vi "Phase control (SubVI).vi"() -> ()   [LabVIEW 2018]
uses:
  <vilib>/measure/mamon.llb/Waveform Peak Detection for 1 Chan.vi
  <vilib>/measure/NI_MAPro.lvlib
panel:
  in  "step search":i32=2 caption="Шаг поиска минимума"
  out "pos_xy":cluster{"pos_x":dbl, "pos_y":dbl} caption="Позиция 2D, мм"
  in  "check":bool
  in  "s_search":bool
  in  "n_search":bool
  in  "start_p_s":bool
  in  "start_p_ns":bool
  out "s_done":bool
  out "n_done":bool
  out "n_sel_pos":dbl
  out "s_sel_pos":dbl
  out "n_arr":dbl[](array[numeric])
  out "s_arr":dbl[](array[numeric])
  in  "input":T1
  out "result":T2
  in  "Go Z":bool
  out "pos_z":dbl caption="Позиция FM"
  in  "К позиции FM":i32
  in  "Шаг, мкм":u32=10000
  in  "Up":bool
  in  "Left":bool
  in  "Down":bool
  in  "Right":bool
  out "error out":errorcluster
  out "pos_s":dbl caption="Уточненное положение\nвыбранного минимума"
  out "pos_n":dbl caption="Уточненное положение\nвыбранного минимума"
  in  "s_sel":dbl=1.0 caption="Порядковый номер \nвыбранного минимума"
  in  "n_sel":dbl=1.0 caption="Порядковый номер \nвыбранного минимума"
  out "s_find":i32 caption="Число мимумов \nна участке (c образцом)"
  out "n_find":i32 caption="Число мимумов \nна участке (без образца)"
  out "Profile_s":cluster{dbl[], dbl[]}(graph) caption="Фазовый профиль (с образцом)"
  out "Profile_ns":cluster{dbl[], dbl[]}(graph) caption="Фазовый профиль (без образца)"
  in  "width":dbl=2.0 caption="Ширина профиля"
  in  "step":i32=10 caption="Шаг сканирования"
  in  "Cancel":bool
  in  "OK":bool
  out "Shown":string
  # "Параметры снятия профиля"
  # "мм"
  # "2D"
  # "мкм"
  # "мкм"
  # "мкм"
  # "мм"
  # "мкм"
  # "N ="
  # "мм"
  # "S ="
  # "мм"
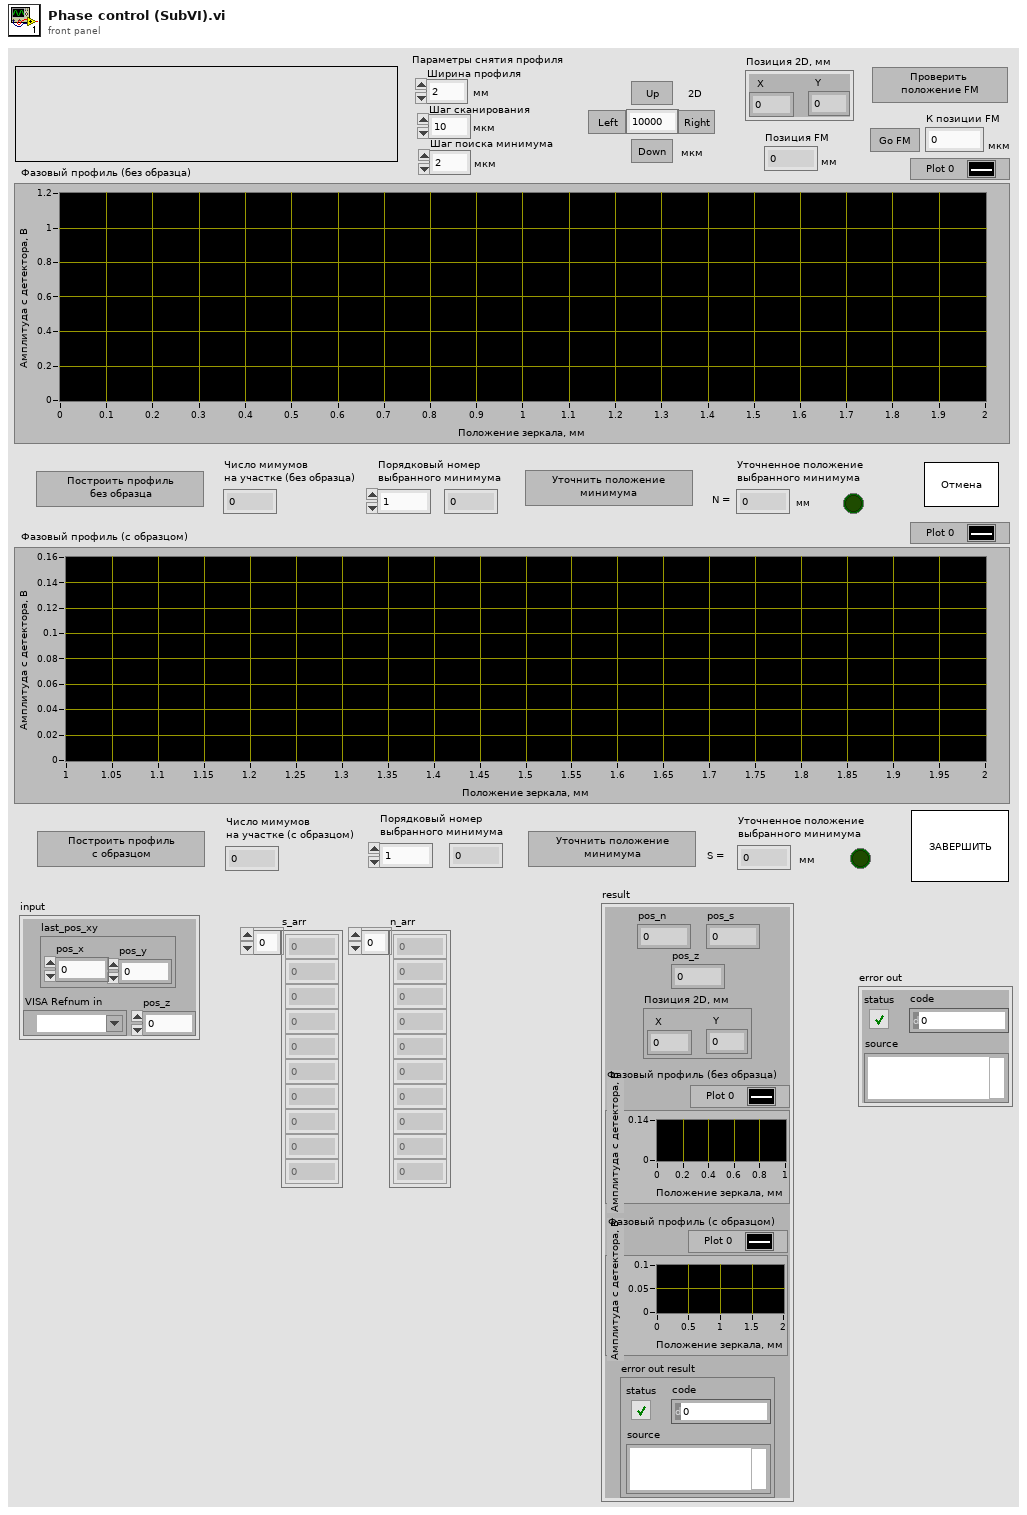
[diagram p1: front panel]
types:
  T1 = cluster{"pos_z":dbl, "VISA Refnum in":refnum<visa-resource-name>, "last_pos_xy":cluster{"pos_x":dbl, "pos_y":dbl}}
  T2 = cluster{"pos_n":dbl, "pos_s":dbl, "pos_z":dbl, "pos_xy 2":cluster{"pos_x":dbl, "pos_y":dbl}, "Profile_ns out":cluster{dbl[], dbl[]}, "Profile_s out":cluster{dbl[], dbl[]}, "error out result":errorcluster}
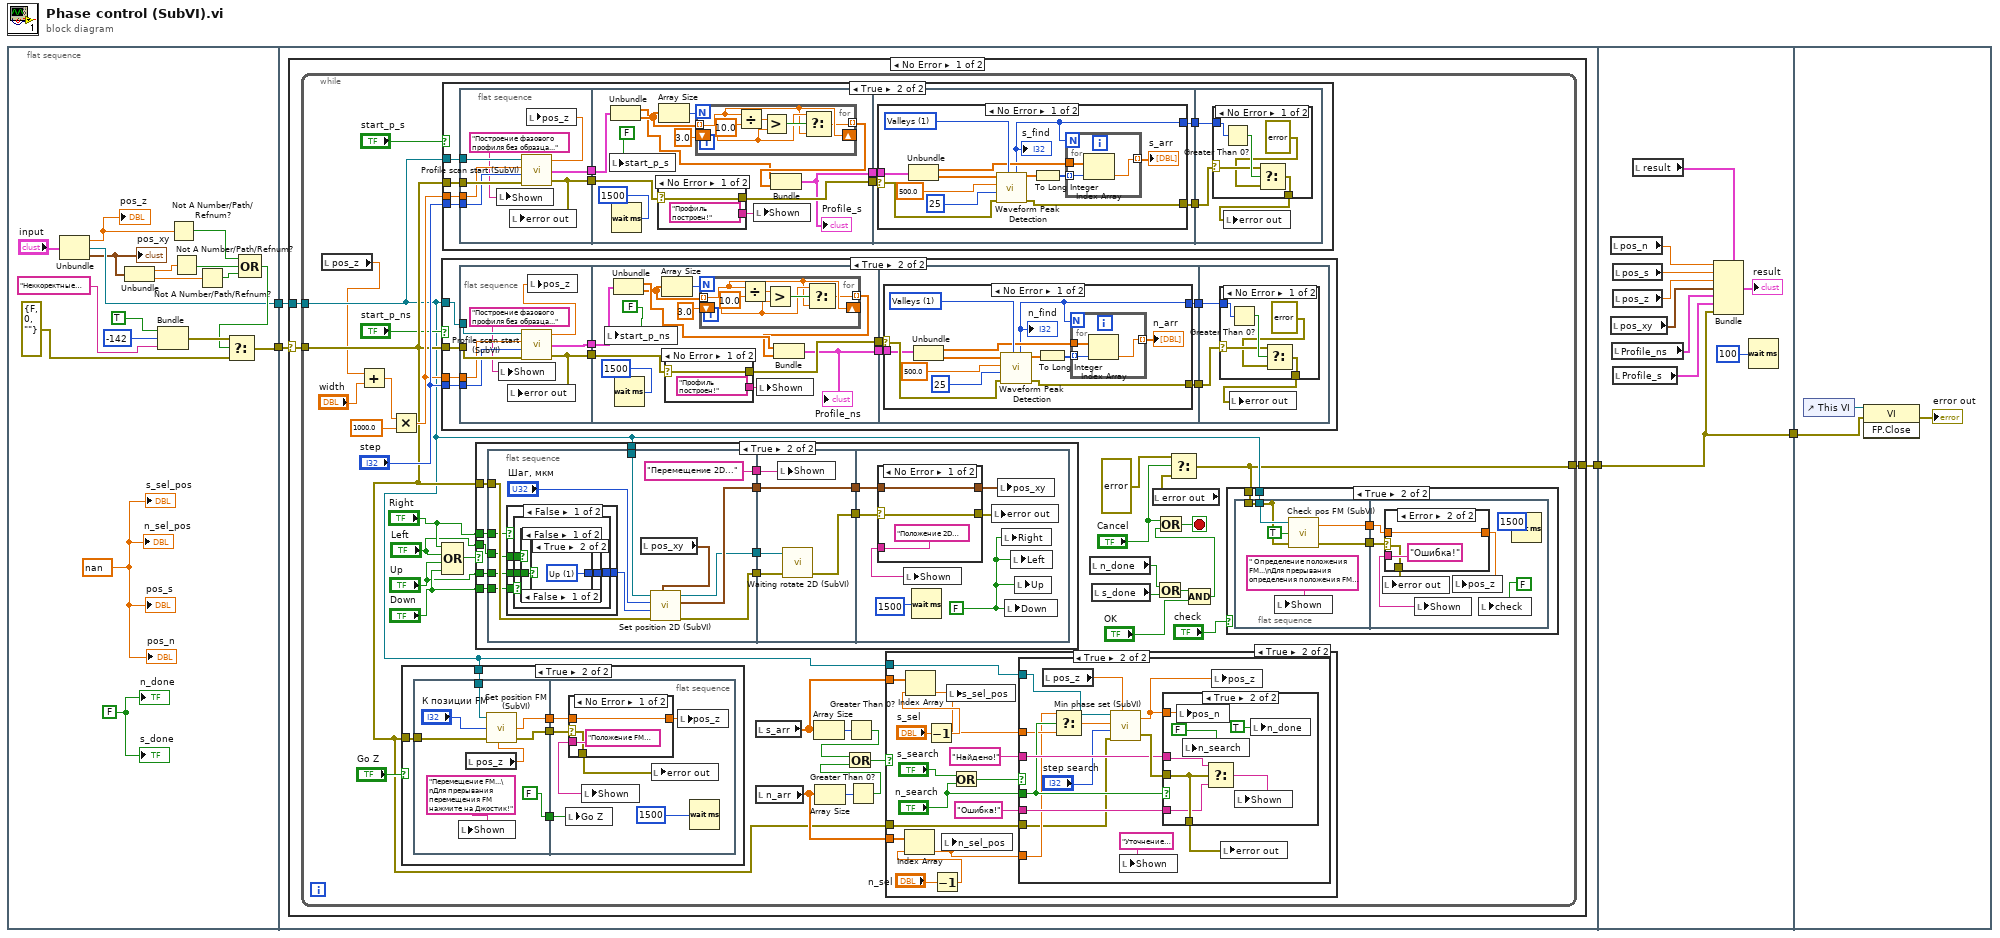
[diagram p0: block diagram]
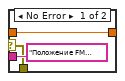
[diagram p3: hidden frame]
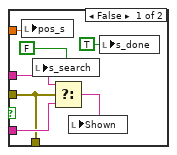
[diagram p6: hidden frame]
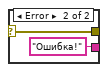
[diagram p8: hidden frame]
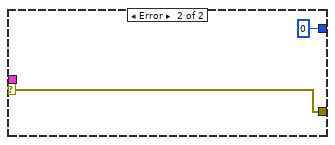
[diagram p9: hidden frame]
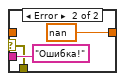
[diagram p12: hidden frame]
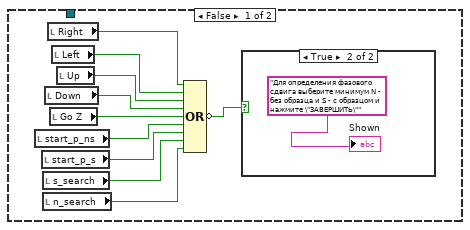
[diagram p13: hidden frame]
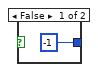
[diagram p15: hidden frame]
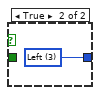
[diagram p16: hidden frame]
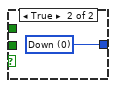
[diagram p17: hidden frame]
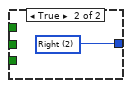
[diagram p18: hidden frame]
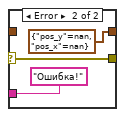
[diagram p19: hidden frame]
diagram:
  n1 = flat-sequence {
    tunnel: [w7] -> w4
    tunnel: [w11] -> w3
    tunnel: w4 -> [w25]
    tunnel: w3 -> [w24]
    tunnel: [w23] -> w2
    tunnel: w2 -> [w364]
    tunnel: [w364] -> w1
    tunnel: w1 -> [w374]
    frame #0 {
      w8 = FALSE ("n_done")
      w9 = nan ("s_sel_pos")
      n2 = Unbundle("input") -> ("pos_z"=w5:dbl, "VISA Refnum in"=w7:refnum<visa-resource-name>, "last_pos_xy"=w6:cluster{"pos_x":dbl, "pos_y":dbl})
      "pos_z" <- w5
      "pos_xy" <- w6
      n3 = Unbundle(w6) -> ("pos_x"=w21:dbl, "pos_y"=w20:dbl)
      n4 = Bundle("status"=TRUE, "code"=-142, "source"="Неккоректные позиции 2D и FM.") -> (w22:errorcluster)  [unwired: 1 in]
      n5 = Not A Number/Path/Refnum?(number/path/refnum=w5) -> (NaN/Path/Refnum?=w19:bool)
      n6 = Not A Number/Path/Refnum?(number/path/refnum=w21) -> (NaN/Path/Refnum?=w18:bool)
      n7 = Not A Number/Path/Refnum?(number/path/refnum=w20) -> (NaN/Path/Refnum?=w17:bool)
      n8 = Compound Arithmetic op=OR(w19, w18, w17) -> (w10:bool)
      n9 = Select(t=w22, s=w10, f=errorcluster {"status"=FALSE, "code"=0, "source"=""} ("t")) -> (s? t:f=w11:errorcluster)
      "pos_n" <- w9
      "pos_s" <- w9
      "s_sel_pos" <- w9
      "n_sel_pos" <- w9
      "s_done" <- w8
      "n_done" <- w8
    }
    frame #1 {
      n10 = case shown="No Error" w24 {
        selector: w24 -> [w27 w363]
        tunnel: w25 -> [w28 _]
        tunnel: [w26 w363] -> w23
        frame No Error {
          n11 = while {
            tunnel: w28 -> [w36]
            tunnel: w27 -> [w45]
            tunnel: [w35] -> w26
            stop <- w56 stop-if-true
            n12 = local read "pos_z"() -> (w32:dbl)
            n13 = Add(x=w32, y="width") -> (x+y=w33:dbl)
            n14 = Multiply(x=w33, y=1000.0) -> (x*y=w47:dbl)
            n15 = case shown="True" "Go Z" {
              tunnel: w36 -> [_ w203]
              tunnel: w45 -> [_ w199]
              frame False {
              }
              frame True {
                n16 = flat-sequence {
                  tunnel: w203 -> [w211]
                  tunnel: w199 -> [w207]
                  tunnel: [w210] -> w202
                  tunnel: [w209] -> w201
                  tunnel: [FALSE ("Rotate FM")] -> w200
                  tunnel: w202 -> [w217]
                  tunnel: w201 -> [w216]
                  tunnel: w200 -> [w213]
                  frame #0 {
                    n17 = local write "Shown"("Перемещение FM...\nДля прерывания перемещения FM нажмите на Джостик!" ("Диалоговое окно")) -> ()
                    n18 = local read "pos_z"() -> (w205:dbl)
                    n19 = call "Set position FM (SubVI).vi"("VISA Refnum in"=w211, "Позиция, мкм"="К позиции FM", "error in"=w207, "pos_z"=w205) -> ("set_pos_z"=w210:dbl, "error out"=w209:errorcluster)  [unwired: 2 in]
                  }
                  frame #1 {
                    n20 = local write "Go Z"(w213) -> ()
                    n21 = case shown="No Error" w216 {
                      selector: w216 -> [w219 w222]
                      tunnel: ["Положение FM достигнуто!" ("Диалоговое окно") "Ошибка!" ("Диалоговое окно")] -> w215
                      tunnel: w217 -> [w220 _]
                      tunnel: [w220 nan ("set_pos_x")] -> w214
                      tunnel: [w219 w222] -> w212
                      frame No Error {
                      }
                      frame Error {
                      }
                    }
                    n22 = local write "Shown"(w215) -> ()
                    n23 = local write "error out"(w212) -> ()
                    n24 = local write "pos_z"(w214) -> ()
                    n25 = Wait (ms)(milliseconds to wait=u32 1500) -> ()  [unwired: 1 out]
                  }
                }
              }
            }
            n26 = case shown="True" "start_p_ns" {
              tunnel: w36 -> [_ w302]
              tunnel: w45 -> [_ w301]
              tunnel: w47 -> [_ w300]
              tunnel: "step" -> [_ w299]
              frame False {
              }
              frame True {
                n27 = flat-sequence {
                  tunnel: w302 -> [w310]
                  tunnel: w301 -> [w309]
                  tunnel: w300 -> [w308]
                  tunnel: w299 -> [w307]
                  tunnel: [w305] -> w298
                  tunnel: [w303] -> w294
                  tunnel: w298 -> [w315]
                  tunnel: [w314] -> w297
                  tunnel: w294 -> [w320]
                  tunnel: [w313] -> w293
                  tunnel: w297 -> [w336]
                  tunnel: [w335] -> w296
                  tunnel: [w334] -> w295
                  tunnel: w293 -> [w333]
                  tunnel: w296 -> [w356]
                  tunnel: w295 -> [w355]
                  frame #0 {
                    n28 = local write "Shown"("Построение фазового профиля без образца..." ("Диалоговое окно")) -> ()
                    n29 = call "Profile scan start (SubVI).vi"("error in"=w309, "Шаг"=w307, "Конец области"=w308, "VISA Refnum in"=w310) -> ("error out"=w305:errorcluster, "Profile"=w303:cluster{dbl[], dbl[]}, "pos_z"=w304:dbl)
                    n30 = local write "error out"(w305) -> ()
                    n31 = local write "pos_z"(w304) -> ()
                  }
                  frame #1 {
                    n32 = local write "start_p_ns"(FALSE ("start p_s")) -> ()
                    n33 = Unbundle(w320) -> (w321:dbl[], w319:dbl[])
                    n34 = Wait (ms)(milliseconds to wait=u32 1500) -> ()  [unwired: 1 out]
                    n35 = Array Size(array=w319) -> (size(s)=w318:i32)
                    n36 = case shown="No Error" w315 {
                      selector: w315 -> [w324 w325]
                      tunnel: ["Профиль построен!" ("Диалоговое окно") "Ошибка!"] -> w311
                      tunnel: [w324 w325] -> w314
                      frame No Error {
                      }
                      frame Error {
                      }
                    }
                    n37 = for {
                      N: w318 -> [_]
                      tunnel: w319 -> [w328] mode=indexing
                      shift-right: [w328] -> _
                      shift-left: 3.0 -> [w329]
                      tunnel: [w327] -> w316 mode=indexing
                      n38 = Divide(x=w328, y=10.0) -> (x/y=w331:dbl)
                      n39 = Greater?(x=w331, y=w329) -> (0:w330:bool)
                      n40 = Select(t=w329, s=w330, f=w328) -> (s? t:f=w327:dbl)
                    }
                    n41 = local write "Shown"(w311) -> ()
                    n42 = Bundle(w321, w316) -> (w313:cluster{dbl[], dbl[]})  [unwired: 1 in]
                    "Profile_ns" <- w313
                  }
                  frame #2 {
                    n43 = case shown="No Error" w336 {
                      selector: w336 -> [w346 w352]
                      tunnel: [w339 0 ("# found")] -> w335
                      tunnel: [w340 w352] -> w334
                      tunnel: w333 -> [w337 _]
                      frame No Error {
                        w348 = u16 1 items=["Peaks", "Valleys"] ("peaks/valleys")
                        n44 = Unbundle(w337) -> (w342:dbl[], w345:dbl[])
                        n45 = call-poly <vilib>:"Waveform Peak Detection.vi"("peaks/valleys"=w348, "error in"=w346, "width"=25, "threshold"=500.0, "Signal In"=w345) -> ("error out"=w340:errorcluster, "Locations"=w344:dbl[], "# found"=w339:i32)  [unwired: 2 in, 2 out]
                        "n_find" <- w339
                        n46 = To Long Integer(number=w344) -> (32bit integer=w343:i32[])
                        n47 = for {
                          N: w339 -> [_]
                          tunnel: w343 -> [w350] mode=indexing
                          tunnel: w342 -> [w351]
                          tunnel: [w349] -> w341 mode=indexing
                          n48 = Index Array(array=w351, index=w350) -> (element=w349:dbl)
                        }
                        "n_arr" <- w341
                      }
                      frame Error {
                      }
                    }
                  }
                  frame #3 {
                    n49 = case shown="No Error" w355 {
                      selector: w355 -> [w359 w362]
                      tunnel: w356 -> [w361 _]
                      tunnel: [w357 w362] -> w354
                      frame No Error {
                        n50 = Greater Than 0?(x=w361) -> (x > 0?=w360:bool)
                        n51 = Select(t=w359, s=w360, f=errorcluster {"status"=TRUE, "code"=-154, "source"="Минимумы не найдены!"} ("error constant")) -> (s? t:f=w357:errorcluster)
                      }
                      frame Error {
                      }
                    }
                    n52 = local write "error out"(w354) -> ()
                  }
                }
              }
            }
            n53 = Compound Arithmetic op=OR("Right", "Left", "Up", "Down") -> (w62:bool)
            n54 = case shown="True" "start_p_s" {
              tunnel: w36 -> [_ w138]
              tunnel: w45 -> [_ w137]
              tunnel: w47 -> [_ w136]
              tunnel: "step" -> [_ w135]
              frame False {
              }
              frame True {
                n55 = flat-sequence {
                  tunnel: w138 -> [w146]
                  tunnel: w137 -> [w145]
                  tunnel: w136 -> [w144]
                  tunnel: w135 -> [w143]
                  tunnel: [w140] -> w134
                  tunnel: [w142] -> w133
                  tunnel: w134 -> [w157]
                  tunnel: w133 -> [w153]
                  tunnel: [w154] -> w132
                  tunnel: [w147] -> w129
                  tunnel: w132 -> [w170]
                  tunnel: [w172] -> w131
                  tunnel: [w171] -> w130
                  tunnel: w129 -> [w169]
                  tunnel: w131 -> [w192]
                  tunnel: w130 -> [w191]
                  frame #0 {
                    n56 = local write "Shown"("Построение фазового профиля без образца..." ("Диалоговое окно")) -> ()
                    n57 = call "Profile scan start (SubVI).vi"("error in"=w145, "Шаг"=w143, "Конец области"=w144, "VISA Refnum in"=w146) -> ("error out"=w140:errorcluster, "Profile"=w142:cluster{dbl[], dbl[]}, "pos_z"=w139:dbl)
                    n58 = local write "error out"(w140) -> ()
                    n59 = local write "pos_z"(w139) -> ()
                  }
                  frame #1 {
                    n60 = local write "start_p_s"(FALSE ("start p_s")) -> ()
                    n61 = Unbundle(w153) -> (w148:dbl[], w150:dbl[])
                    n62 = Wait (ms)(milliseconds to wait=u32 1500) -> ()  [unwired: 1 out]
                    n63 = case shown="No Error" w157 {
                      selector: w157 -> [w165 w167]
                      tunnel: ["Профиль построен!" ("Диалоговое окно") "Ошибка!"] -> w158
                      tunnel: [w165 w167] -> w154
                      frame No Error {
                      }
                      frame Error {
                      }
                    }
                    n64 = Array Size(array=w150) -> (size(s)=w151:i32)
                    n65 = for {
                      N: w151 -> [_]
                      tunnel: w150 -> [w160] mode=indexing
                      shift-right: [w160] -> _
                      shift-left: 3.0 -> [w161]
                      tunnel: [w159] -> w149 mode=indexing
                      n66 = Divide(x=w160, y=10.0) -> (x/y=w163:dbl)
                      n67 = Greater?(x=w163, y=w161) -> (0:w162:bool)
                      n68 = Select(t=w161, s=w162, f=w160) -> (s? t:f=w159:dbl)
                    }
                    n69 = local write "Shown"(w158) -> ()
                    n70 = Bundle(w148, w149) -> (w147:cluster{dbl[], dbl[]})  [unwired: 1 in]
                    "Profile_s" <- w147
                  }
                  frame #2 {
                    n71 = case shown="No Error" w170 {
                      selector: w170 -> [w182 w188]
                      tunnel: [w176 0 ("# found")] -> w172
                      tunnel: [w175 w188] -> w171
                      tunnel: w169 -> [w173 _]
                      frame No Error {
                        w184 = u16 1 items=["Peaks", "Valleys"] ("peaks/valleys")
                        n72 = Unbundle(w173) -> (w178:dbl[], w181:dbl[])
                        n73 = call-poly <vilib>:"Waveform Peak Detection.vi"("peaks/valleys"=w184, "error in"=w182, "width"=25, "threshold"=500.0, "Signal In"=w181) -> ("error out"=w175:errorcluster, "Locations"=w180:dbl[], "# found"=w176:i32)  [unwired: 2 in, 2 out]
                        "s_find" <- w176
                        n74 = To Long Integer(number=w180) -> (32bit integer=w179:i32[])
                        n75 = for {
                          N: w176 -> [_]
                          tunnel: w179 -> [w186] mode=indexing
                          tunnel: w178 -> [w187]
                          tunnel: [w185] -> w177 mode=indexing
                          n76 = Index Array(array=w187, index=w186) -> (element=w185:dbl)
                        }
                        "s_arr" <- w177
                      }
                      frame Error {
                      }
                    }
                  }
                  frame #3 {
                    n77 = case shown="No Error" w191 {
                      selector: w191 -> [w195 w198]
                      tunnel: w192 -> [w197 _]
                      tunnel: [w193 w198] -> w190
                      frame No Error {
                        n78 = Greater Than 0?(x=w197) -> (x > 0?=w196:bool)
                        n79 = Select(t=w195, s=w196, f=errorcluster {"status"=TRUE, "code"=-154, "source"="Минимумы не найдены!"} ("error constant")) -> (s? t:f=w193:errorcluster)
                      }
                      frame Error {
                      }
                    }
                    n80 = local write "error out"(w190) -> ()
                  }
                }
              }
            }
            n81 = case shown="True" w62 {
              tunnel: w36 -> [_ w247]
              tunnel: w45 -> [_ w246]
              tunnel: "Right" -> [_ w239]
              tunnel: "Down" -> [_ w238]
              tunnel: "Left" -> [_ w237]
              tunnel: "Up" -> [_ w236]
              frame False {
                n82 = local read "start_p_ns"() -> (w228:bool)
                n83 = local read "start_p_s"() -> (w227:bool)
                n84 = local read "s_search"() -> (w226:bool)
                n85 = local read "n_search"() -> (w225:bool)
                n86 = local read "Down"() -> (w230:bool)
                n87 = local read "Right"() -> (w233:bool)
                n88 = local read "Go Z"() -> (w229:bool)
                n89 = local read "Left"() -> (w232:bool)
                n90 = local read "Up"() -> (w231:bool)
                n91 = Compound Arithmetic op=OR(w233, w232, w231, w230, w229, w228, w227, w226, w225) -> (invert w234:bool)
                n92 = case shown="True" w234 {
                  frame False {
                  }
                  frame True {
                    "Shown" <- "Для определения фазового сдвига выберите минимум N - без образца и S - с образцом и нажмите \"ЗАВЕРШИТЬ\"" ("Prompt (system name provided)")
                  }
                }
              }
              frame True {
                n93 = flat-sequence {
                  tunnel: w247 -> [w251]
                  tunnel: w246 -> [w260]
                  tunnel: [w259] -> w244
                  tunnel: ["Перемещение 2D..." ("Диалоговое окно")] -> w242
                  tunnel: [w257] -> w241
                  tunnel: [w256] -> w240
                  tunnel: w239 -> [w255]
                  tunnel: w238 -> [w254]
                  tunnel: w237 -> [w253]
                  tunnel: w236 -> [w252]
                  tunnel: [w276] -> w245
                  tunnel: w244 -> [w279]
                  tunnel: [w279] -> w243
                  tunnel: w242 -> [w278]
                  tunnel: w241 -> [w277]
                  tunnel: w240 -> [w275]
                  tunnel: w245 -> [w285]
                  tunnel: w243 -> [w284]
                  frame #0 {
                    n94 = case shown="False" w255 {
                      tunnel: w254 -> [w264 _]
                      tunnel: [w263 w274] -> w250
                      tunnel: w253 -> [w262 _]
                      tunnel: w252 -> [w261 _]
                      frame False {
                        n95 = case shown="False" w264 {
                          tunnel: [w266 w273] -> w263
                          tunnel: w262 -> [w267 _]
                          tunnel: w261 -> [w265 _]
                          frame False {
                            n96 = case shown="False" w267 {
                              tunnel: [w268 w272] -> w266
                              tunnel: w265 -> [w269 _]
                              frame False {
                                n97 = case shown="True" w269 {
                                tunnel: [-1 w271] -> w268
                                frame False {
                                }
                                frame True {
                                w271 = u16 1 items=["Down", "Up", "Right", "Left"] ("Direct")
                                }
                                }
                              }
                              frame True {
                                w272 = u16 3 items=["Down", "Up", "Right", "Left"] ("Direct")
                              }
                            }
                          }
                          frame True {
                            w273 = u16 0 items=["Down", "Up", "Right", "Left"] ("Direct")
                          }
                        }
                      }
                      frame True {
                        w274 = u16 2 items=["Down", "Up", "Right", "Left"] ("Direct")
                      }
                    }
                    n98 = local read "pos_xy"() -> (w249:cluster{"pos_x":dbl, "pos_y":dbl})
                    n99 = call "Set position 2D (SubVI).vi"("last_pos_xy"=w249, "error in"=w260, "Direct"=w250, "Шаг"="Шаг, мкм", "VISA Refnum in"=w251) -> ("error out"=w257:errorcluster, "set_pos_xy"=w259:cluster{"pos_x":dbl, "pos_y":dbl}, "VISA Refnum out"=w256:refnum<visa-resource-name>)  [unwired: 2 in]
                  }
                  frame #1 {
                    n100 = local write "Shown"(w278) -> ()
                    n101 = call "Waiting rotate 2D (SubVI).vi"("error in (no error)"=w277, "VISA Refnum in"=w275) -> ("error out"=w276:errorcluster)  [unwired: 3 in]
                  }
                  frame #2 {
                    w283 = FALSE ("Go 2D")
                    n102 = case shown="No Error" w285 {
                      selector: w285 -> [w288 w291]
                      tunnel: ["Положение 2D достигнуто!" ("Диалоговое окно") "Ошибка!" ("Диалоговое окно")] -> w281
                      tunnel: w284 -> [w287 _]
                      tunnel: [w288 w291] -> w280
                      tunnel: [w287 cluster{"pos_y":dbl, "pos_x":dbl} {"pos_y"=nan, "pos_x"=nan} ("set_pos_xy")] -> w282
                      frame No Error {
                      }
                      frame Error {
                      }
                    }
                    n103 = local write "Shown"(w281) -> ()
                    n104 = Wait (ms)(milliseconds to wait=u32 1500) -> ()  [unwired: 1 out]
                    n105 = local write "error out"(w280) -> ()
                    n106 = local write "pos_xy"(w282) -> ()
                    n107 = local write "Right"(w283) -> ()
                    n108 = local write "Down"(w283) -> ()
                    n109 = local write "Left"(w283) -> ()
                    n110 = local write "Up"(w283) -> ()
                  }
                }
              }
            }
            n111 = local read "s_arr"() -> (w49:dbl[])
            n112 = local read "n_arr"() -> (w50:dbl[])
            n113 = Array Size(array=w49) -> (size(s)=w55:i32)
            n114 = Array Size(array=w50) -> (size(s)=w54:i32)
            n115 = Greater Than 0?(x=w55) -> (x > 0?=w52:bool)
            n116 = Greater Than 0?(x=w54) -> (x > 0?=w51:bool)
            n117 = Or(x=w52, y=w51) -> (x .or. y?=w53:bool)
            n118 = case shown="True" w53 {
              tunnel: w50 -> [_ w96]
              tunnel: w49 -> [_ w100]
              tunnel: w36 -> [_ w90]
              tunnel: w45 -> [_ w94]
              frame False {
              }
              frame True {
                n119 = Decrement(x="s_sel") -> (x-1=w93:dbl)
                n120 = Index Array(array=w100, index=w93) -> (element=w87:dbl)
                n121 = Decrement(x="n_sel") -> (x-1=w98:dbl)
                n122 = Index Array(array=w96, index=w98) -> (element=w86:dbl)
                n123 = local write "n_sel_pos"(w86) -> ()
                n124 = local write "s_sel_pos"(w87) -> ()
                n125 = Or(x="s_search", y="n_search") -> (x .or. y?=w95:bool)
                n126 = case shown="True" w95 {
                  tunnel: w94 -> [_ w101]
                  tunnel: w90 -> [_ w103]
                  tunnel: "n_search" -> [_ w108]
                  tunnel: "Найдено!" ("Shown") -> [_ w112]
                  tunnel: "Ошибка!" ("Shown") -> [_ w111]
                  tunnel: w87 -> [_ w107]
                  tunnel: w86 -> [_ w106]
                  frame False {
                  }
                  frame True {
                    n127 = local read "pos_z"() -> (w109:dbl)
                    n128 = Select(t=w106, s=w108, f=w107) -> (s? t:f=w105:dbl)
                    n129 = call "Min phase set (SubVI).vi"("pos_z"=w109, "error in"=w101, "step search"="step search", "set_pos_min"=w105, "VISA Refnum in"=w103) -> ("error out"=w113:errorcluster, "Min phase"=w104:dbl)  [unwired: 1 in]
                    n130 = local write "Shown"("Уточнение положения минимума фазы..." ("Shown")) -> ()
                    n131 = case shown="True" w108 {
                      tunnel: w104 -> [w121 w128]
                      tunnel: w113 -> [w115 w125]
                      tunnel: w112 -> [w118 w124]
                      tunnel: w111 -> [w117 w123]
                      tunnel: [w115 w125] -> w110
                      frame False {
                        n132 = local write "pos_s"(w121) -> ()
                        n133 = local write "s_search"(FALSE) -> ()
                        n134 = Select(t=w118, s=w115, f=w117) -> (s? t:f=w116:string)
                        n135 = local write "Shown"(w116) -> ()
                        n136 = local write "s_done"(TRUE) -> ()
                      }
                      frame True {
                        n137 = local write "pos_n"(w128) -> ()
                        n138 = local write "n_search"(FALSE) -> ()
                        n139 = Select(t=w124, s=w125, f=w123) -> (s? t:f=w122:string)
                        n140 = local write "Shown"(w122) -> ()
                        n141 = local write "n_done"(TRUE ("n_done")) -> ()
                      }
                    }
                    n142 = local write "pos_z"(w104) -> ()
                    n143 = local write "error out"(w110) -> ()
                  }
                }
              }
            }
            n144 = local read "n_done"() -> (w31:bool)
            n145 = local read "s_done"() -> (w30:bool)
            n146 = local read "error out"() -> (w43:errorcluster)
            n147 = Or(x=w31, y=w30) -> (x .or. y?=w29:bool)
            n148 = Select(t=errorcluster {"status"=TRUE, "code"=-1, "source"="Отмена построения профиля!"} ("error constant"), s="Cancel", f=w43) -> (s? t:f=w35:errorcluster)
            n149 = Compound Arithmetic op=AND(w29, "OK") -> (w40:bool)
            n150 = Or(x="Cancel", y=w40) -> (x .or. y?=w56:bool)
            n151 = case shown="True" "check" {
              tunnel: w36 -> [_ w64]
              tunnel: w35 -> [_ w63]
              frame False {
              }
              frame True {
                n152 = flat-sequence {
                  tunnel: w64 -> [w72]
                  tunnel: [w67] -> _
                  tunnel: [w71] -> w66
                  tunnel: [w70] -> w65
                  tunnel: w63 -> [w67]
                  tunnel: w66 -> [w79]
                  tunnel: w65 -> [w78]
                  frame #0 {
                    n153 = local write "Shown"(" Определение положения FM...\nДля прерывания определения положения FM нажмите на Джостик!" ("Диалоговое окно")) -> ()
                    n154 = call "Check pos FM (SubVI).vi"("error in"=w67, "verify?"=TRUE, "VISA Refnum in"=w72) -> ("error out"=w71:errorcluster, "position"=w70:dbl)
                  }
                  frame #1 {
                    n155 = case shown="Error" w79 {
                      selector: w79 -> [w81 w84]
                      tunnel: ["Положение FM определено!" ("Диалоговое окно") "Ошибка!" ("Диалоговое окно")] -> w76
                      tunnel: [w80 w83] -> w77
                      tunnel: [w81 w84] -> w73
                      tunnel: w78 -> [w80 w83]
                      frame No Error {
                      }
                      frame Error {
                      }
                    }
                    n156 = local write "error out"(w73) -> ()
                    n157 = local write "Shown"(w76) -> ()
                    n158 = local write "pos_z"(w77) -> ()
                    n159 = local write "check"(FALSE) -> ()
                    n160 = Wait (ms)(milliseconds to wait=u32 1500) -> ()  [unwired: 1 out]
                  }
                }
              }
            }
          }
        }
        frame Error {
        }
      }
    }
    frame #2 {
      n161 = local read "pos_n"() -> (w373:dbl)
      n162 = local read "pos_xy"() -> (w368:cluster{"pos_x":dbl, "pos_y":dbl})
      n163 = local read "Profile_ns"() -> (w366:cluster{dbl[], dbl[]})
      n164 = local read "pos_s"() -> (w372:dbl)
      n165 = local read "pos_z"() -> (w371:dbl)
      n166 = local read "Profile_s"() -> (w365:cluster{dbl[], dbl[]})
      n167 = local read "result"() -> (w369:T2)
      n168 = Bundle(cluster=w369, "pos_n"=w373, "pos_s"=w372, "pos_z"=w371, "pos_xy 2"=w368, "Profile_ns out"=w366, "Profile_s out"=w365, "error out result"=w364) -> (→"result":T2)
      n169 = Wait (ms)(milliseconds to wait=u32 100) -> ()  [unwired: 1 out]
    }
    frame #3 {
      n170 = control-ref of="This VI"() -> (w375:refnum<vi>)
      n171 = invoke class="VI" method="FP.Close"(reference=w375, error in=w374) -> (error out=→"error out":errorcluster)  [unwired: 1 in, 2 out]
    }
  }
